vi "PrepareMetadaDataForDisplay.vi"(0 "MeasurementMetadata":string[][](array[string])) -> (1 "String array":string[](array[string]))   [LabVIEW 2017]
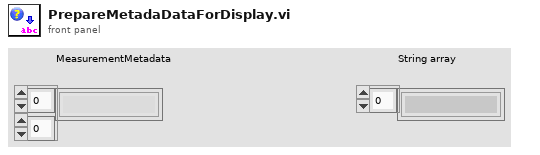
[diagram p1: front panel]
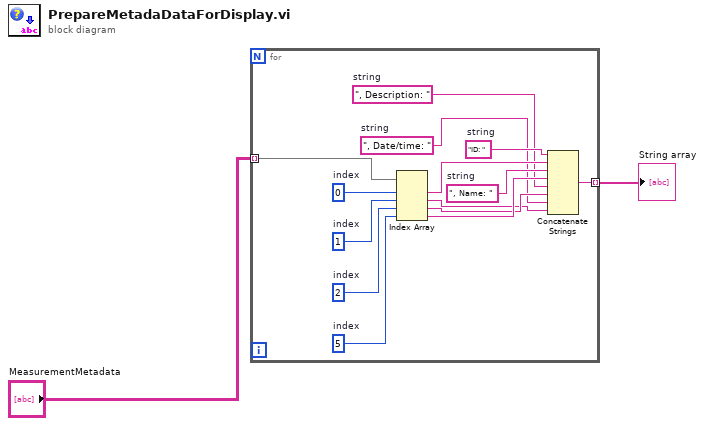
[diagram p0: block diagram]
diagram:
  n1 = for {
    tunnel: "MeasurementMetadata" -> [w16] mode=indexing
    tunnel: [w11] -> w1 mode=indexing
    w4 = ", Date/time: "  # string
    w6 = ", Description: "  # string
    w8 = ", Name: "  # string
    w10 = "ID: "  # string
    w12 = 5  # index
    w13 = 2  # index
    w14 = 1  # index
    w15 = 0  # index
    n2 = Index Array(array=w16, index #1=w15, index #2=w14, index #3=w13, index #4=w12) -> (element #1=w9:string, element #2=w3:string, element #3=w5:string, element #4=w7:string)
    n3 = Concatenate Strings(w10, w9, w8, w7, w6, w5, w4, w3) -> (w11:string)
  }
  "String array" <- w1
